vi "Entry Initialize (User).vi"(8 "error in":errorcluster, 11 "Node in":refnum<class "BLS Power Supply Template.lvclass">) -> (0 "error out":errorcluster, 3 "Node out":refnum<class "BLS Power Supply Template.lvclass">)   [LabVIEW 2023, in "BLS Power Supply Template.lvlib" / "BLS Power Supply Template.lvclass"]
uses:
  BLS Power Supply Template.lvclass
  BLS Power Supply Template.lvclass/BLS Power Supply Template.ctl
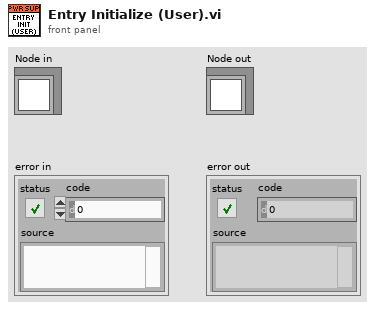
[diagram p1: front panel]
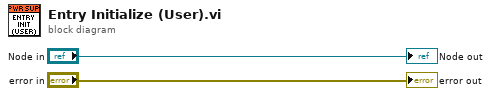
[diagram p0: block diagram]
diagram:
  "Node out" <- "Node in"
  "error out" <- "error in"
